vi "Main.vi"(8 "error in":errorcluster, 11 "subWorker Level 2 in":refnum<class "subWorker Level 2.lvclass">) -> (0 "error out":errorcluster, 3 "subWorker Level 2 out":refnum<class "subWorker Level 2.lvclass">)   [LabVIEW 2017, in "subWorker Level 2.lvclass"]
doc: "The <b>Queued Message Handler</b> of the Worker that owns this VI."
uses:
  subWorker Level 2.lvclass
  Initialization Data.ctl
  Response Cases.ctl
  subWorker Level 2.lvclass/subWorker Level 2.ctl
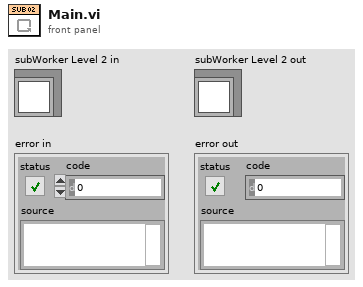
[diagram p1: front panel]
types:
  T1 = typedef "subWorker Level 2.lvclass/Initialization Data.ctl" = cluster{"Response Cases":T2}
  T2 = typedef "subWorker Level 2.lvclass/Response Cases.ctl" = cluster{"Placeholder - Can be deleted":string}
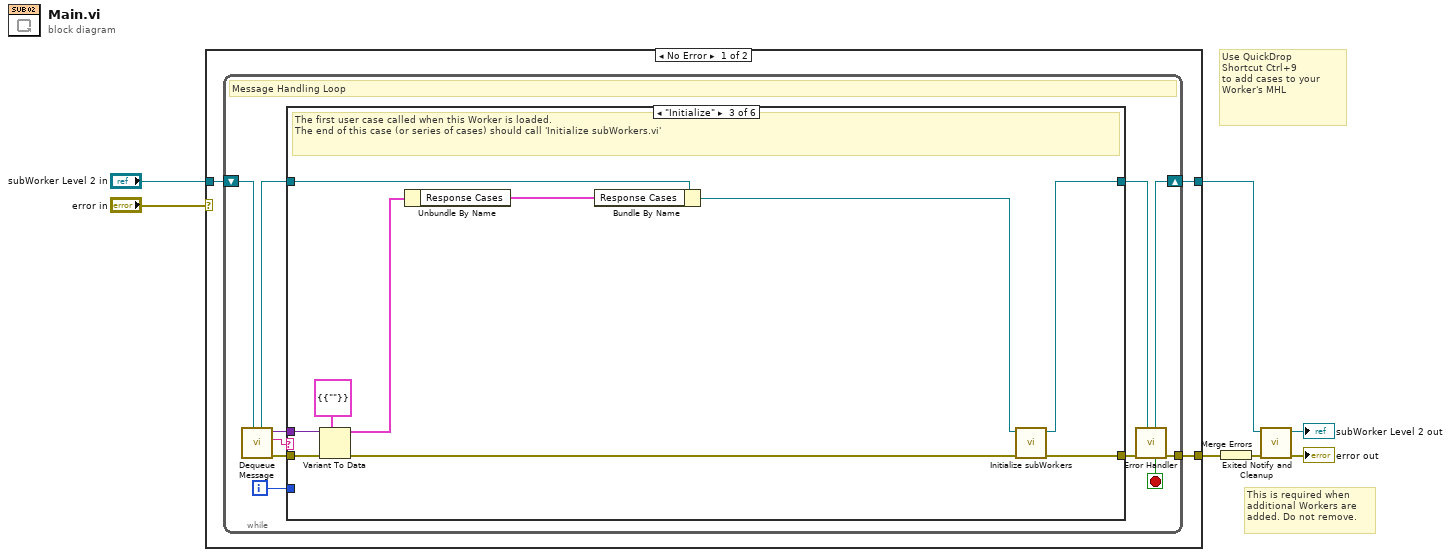
[diagram p0: block diagram]
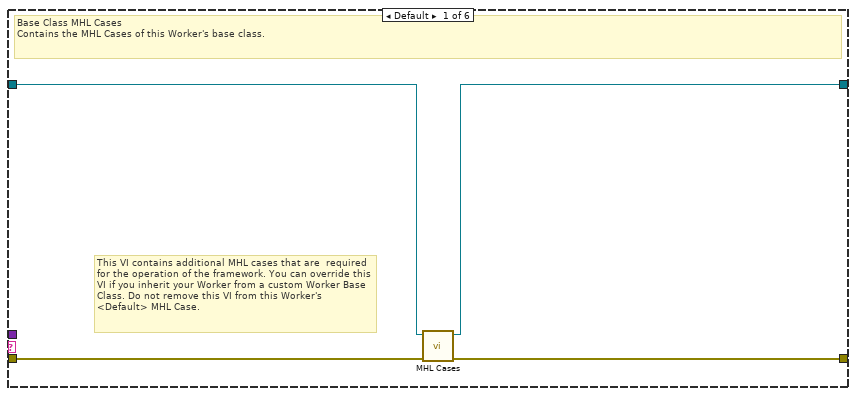
[diagram p2: hidden frame]
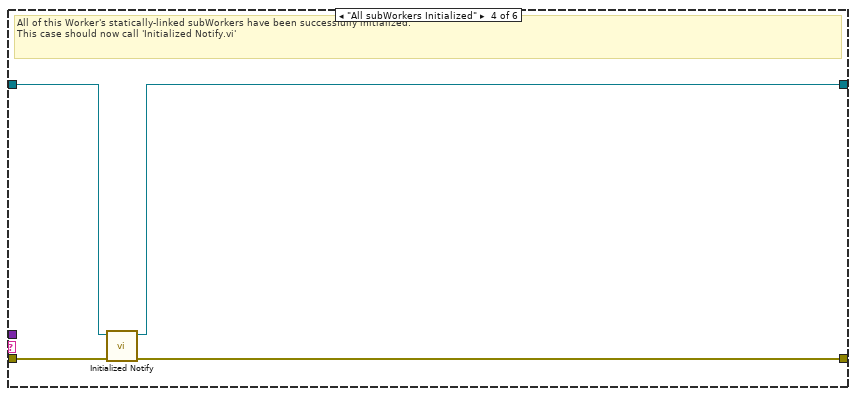
[diagram p4: hidden frame]
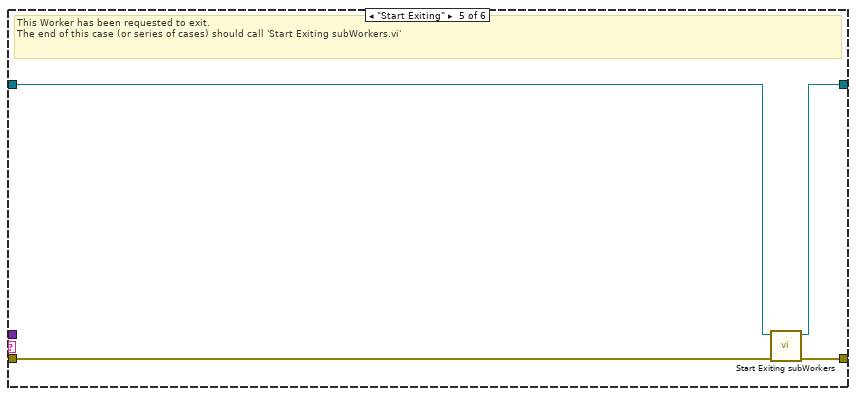
[diagram p5: hidden frame]
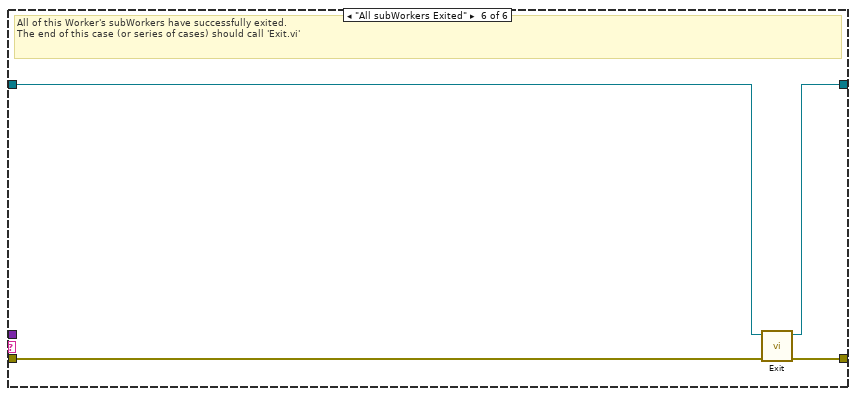
[diagram p6: hidden frame]
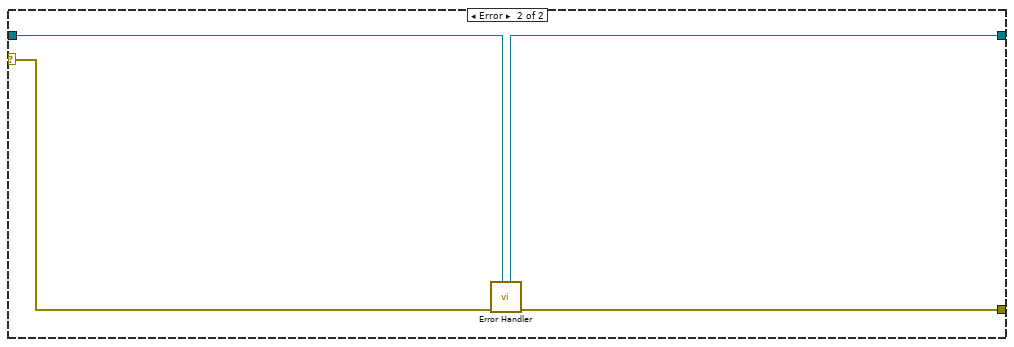
[diagram p7: hidden frame]
diagram:
  # "Use QuickDrop\nShortcut Ctrl+9\nto add cases to your\nWorker's MHL"
  # "This is required when additional Workers are added. Do not remove."
  n1 = case shown="No Error" "error in" {
    tunnel: "subWorker Level 2 in" -> [w8 w51]
    tunnel: [w10 w52] -> w6
    tunnel: [w9 w50] -> w7
    selector: "error in" -> [_ w53]
    frame No Error {
      n2 = while {
        shift-right: [w19] -> w9
        shift-left: w8 -> [w21]
        tunnel: [w20] -> w10
        i -> [w11]
        stop <- w12 stop-if-true
        # "Message Handling Loop"
        n3 = call-dynamic "Dequeue Message.vi"("Worker"=w21) -> ("error out"=w18:errorcluster, "Case out"=w13:string, "Data out"=w14:variant, "Worker out"=w16:refnum<class "subWorker Level 2.lvclass">)  [unwired: 6 in, 1 out]
        n4 = case "Worker MHL Case Structure (DO NOT CHANGE LABEL NAME)" shown="\"Initialize\"" w13 {
          tunnel: w18 -> [w25 w26 w35 w41 w42 w49]
          tunnel: [w24 w26 w37 w40 w45 w48] -> w17
          tunnel: w16 -> [w23 w27 w34 w39 w43 w47]
          tunnel: [w22 w27 w36 w38 w44 w46] -> w15
          tunnel: w14 -> [_ _ w32 _ _ _]
          tunnel: w11 -> [_ _ _ _ _ _]
          frame Default {
            # "This VI contains additional MHL cases that are  required for the operation of the framework. You can override this VI if you inherit your Worker from a custom Worker Base Class. Do not remove this VI from this Worker's <Default> MHL Case."
            # "Base Class MHL Cases\nContains the MHL Cases of this Worker's base class."
            n5 = call-dynamic "MHL Cases.vi"("error in"=w25, "Worker Base Class in"=w23) -> ("error out"=w24:errorcluster, "Worker Base Class out"=w22:refnum<class "subWorker Level 2.lvclass">)  [unwired: 8 in]
          }
          frame "------------ FRAMEWORK CASES -----------" {
            # "Start of Workers Framework Cases"
          }
          frame "Initialize" {
            # "The first user case called when this Worker is loaded.\nThe end of this case (or series of cases) should call 'Initialize subWorkers.vi'"
            n6 = Variant To Data(error in=w35, type=T1 {"Response Cases"={"Placeholder - Can be deleted"=""}} ("Cluster"), Variant=w32) -> (data=w31:T1, error out=w33:errorcluster)
            n7 = Unbundle By Name(w31) -> ("Response Cases"=w30:T2)
            n8 = Bundle By Name(cluster=w34, "Response Cases"=w30) -> (w28:refnum<class "subWorker Level 2.lvclass">)
            n9 = call-dynamic "Initialize subWorkers.vi"("error in"=w33, "Worker"=w28) -> ("error out"=w37:errorcluster, "dup Worker out"=w36:refnum<class "subWorker Level 2.lvclass">)  [unwired: 8 in]
          }
          frame "All subWorkers Initialized" {
            # "All of this Worker's statically-linked subWorkers have been successfully initialized.\nThis case should now call 'Initialized Notify.vi'"
            n10 = call-dynamic "Initialized Notify.vi"("error in"=w41, "Worker"=w39) -> ("error out"=w40:errorcluster, "dup Worker out"=w38:refnum<class "subWorker Level 2.lvclass">)  [unwired: 8 in]
          }
          frame "Start Exiting" {
            # "This Worker has been requested to exit. \nThe end of this case (or series of cases) should call 'Start Exiting subWorkers.vi'"
            n11 = call-dynamic "Start Exiting subWorkers.vi"("error_in"=w42, "Worker"=w43) -> ("error out"=w45:errorcluster, "dup Worker out"=w44:refnum<class "subWorker Level 2.lvclass">)  [unwired: 8 in]
          }
          frame "All subWorkers Exited" {
            # "All of this Worker's subWorkers have successfully exited. \nThe end of this case (or series of cases) should call 'Exit.vi'"
            n12 = call-dynamic "Exit.vi"("error_in"=w49, "Worker"=w47) -> ("error out"=w48:errorcluster, "dup Worker out"=w46:refnum<class "subWorker Level 2.lvclass">)  [unwired: 8 in]
          }
        }
        n13 = call-dynamic "Error Handler.vi"("Worker"=w15, "error_in"=w17) -> ("error out"=w20:errorcluster, "Stop Loop"=w12:bool, "Worker out"=w19:refnum<class "subWorker Level 2.lvclass">)  [unwired: 7 in]
      }
    }
    frame Error {
      n14 = call-dynamic "Error Handler.vi"("Worker"=w51, "error_in"=w53) -> ("error out"=w52:errorcluster, "Worker out"=w50:refnum<class "subWorker Level 2.lvclass">)  [unwired: 7 in, 1 out]
    }
  }
  n15 = Merge Errors(w6) -> (w3:errorcluster)
  n16 = call-dynamic "Exited Notify and Cleanup.vi"("error_in"=w3, "Worker"=w7) -> ("error out"=→"error out":errorcluster, "dup Worker out"=→"subWorker Level 2 out":refnum<class "subWorker Level 2.lvclass">)  [unwired: 8 in]
